vi "Get All Endpoint Configurations.vi"(8 "error in":errorcluster, 11 "endpoint configuration in":T3 format="%.0x") -> (0 "error out":errorcluster, 2 "endpoint configurations":T1[](array[typedef]), 3 "endpoint configuration out":T3 format="%.0x")   [LabVIEW 2017, in "NI-SWITCH Scripting.lvlib"]
doc: "Returns the configuration for all endpoints."
uses:
  NI-SWITCH Scripting.lvlib
  <vilib>/NI Veristand/Custom Device API/Custom Device Item Ref.ctl
  Shared/Endpoint Configuration Cluster.ctl
  Shared/Endpoint Configuration Enum.ctl
  <vilib>/NI VeriStand/Custom Device API/Custom Device API.lvlib
  Shared/NI-SWITCH Shared.lvlib
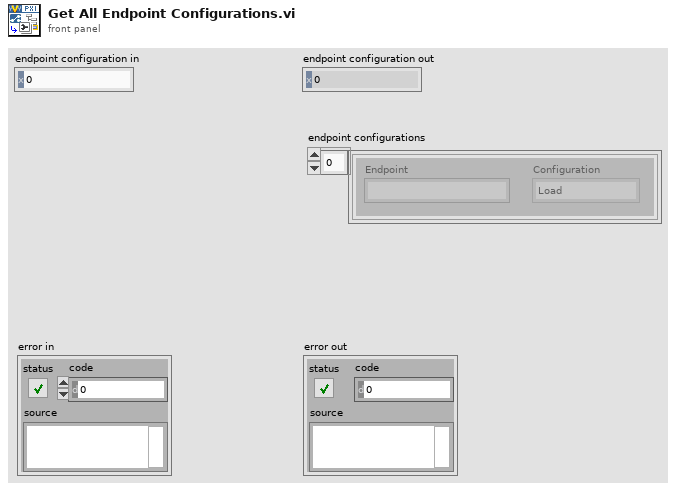
[diagram p1: front panel]
types:
  T1 = typedef "NI-SWITCH Shared.lvlib/Endpoint Configuration Cluster.ctl" = cluster{"Endpoint":string, "Configuration":T2}
  T2 = typedef "NI-SWITCH Shared.lvlib/Endpoint Configuration Enum.ctl" = enum16{"Load", "Source", "Configuration"}
  T3 = typedef "Custom Device API.lvlib/Custom Device Item Ref.ctl" = u64
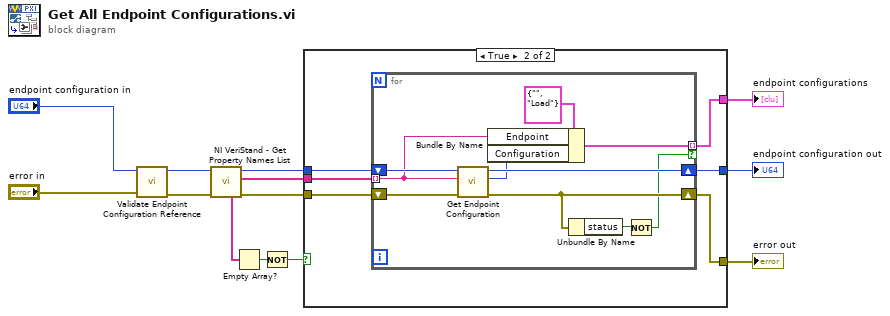
[diagram p0: block diagram]
diagram:
  n1 = call "Validate Endpoint Configuration Reference.vi"("error in"="error in", "endpoint configuration in"="endpoint configuration in") -> ("error out"=w3:errorcluster, "endpoint configuration out"=w2:T3)  [unwired: 8 in]
  n2 = call <vilib>:"NI VeriStand - Get Property Names List.vi"("error in (no error)"=w3, "Item Ref in"=w2) -> ("error out"=w10:errorcluster, "Property Names"=w11:string[], "Item Ref out"=w6:T3)  [unwired: 7 in]
  n3 = Empty Array?(array=w11) -> (empty?=w12:bool)
  n4 = Not(x=w12) -> (.not. x?=w4:bool)
  n5 = case shown="True" w4 {
    tunnel: w11 -> [_ w20]
    tunnel: w10 -> [w13 w19]
    tunnel: [_ w18] -> w8
    tunnel: [w13 w17] -> w7
    tunnel: w6 -> [w14 w16]
    tunnel: [w14 w15] -> w5
    frame False {
    }
    frame True {
      n6 = for {
        tunnel: w20 -> [w26] mode=indexing
        shift-right: [w23] -> w17
        shift-left: w19 -> [w27]
        tunnel: [w30] -> w18 mode=indexing if=w21
        shift-right: [w28] -> w15
        shift-left: w16 -> [w29]
        n7 = call "Get Endpoint Configuration.vi"("error in"=w27, "endpoint"=w26, "endpoint configuration in"=w29) -> ("error out"=w23:errorcluster, "configuration"=w25:T2, "endpoint configuration out"=w28:T3)  [unwired: 6 in]
        n8 = Bundle By Name(cluster=T1 {"Endpoint"="", "Configuration"=enum."Load"} ("Connection"), "Endpoint"=w26, "Configuration"=w25) -> (w30:T1)
        n9 = Unbundle By Name(w23) -> ("status"=w22:bool)
        n10 = Not(x=w22) -> (.not. x?=w21:bool)
      }
    }
  }
  "error out" <- w7
  "endpoint configuration out" <- w5
  "endpoint configurations" <- w8
